vi "Rack Status.vi"(7 "Address":u16, 8 "Error In":errorcluster, 11 "VISA Resource in":refnum<visa-resource-name>) -> (0 "Error Out":errorcluster, 1 "Rack Status Cluster":T1, 2 "Rack Status":u8 format="%.0b", 3 "VISA Resource out":refnum<visa-resource-name>)   [LabVIEW 2015, in "KIT QV.lvlib"]
doc: "Read rack status. It's the OR/AND of all marked detectors including status of control mode."
uses:
  KIT QV.lvlib
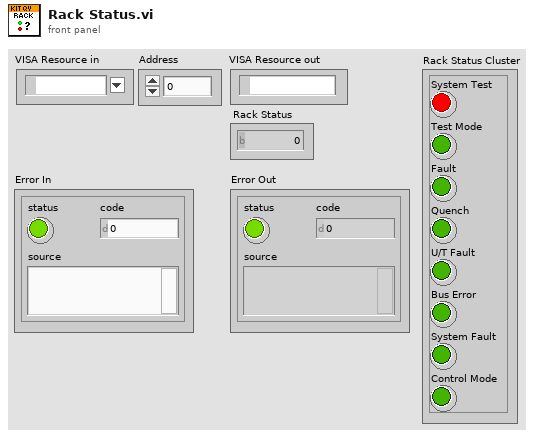
[diagram p1: front panel]
types:
  T1 = cluster{"System Test":bool, "Test Mode":bool, "Fault":bool, "Quench":bool, "U/T Fault":bool, "Bus Error":bool, "System Fault":bool, "Control Mode":bool}
  T2 = cluster{"Boolean array[0]":bool, "Boolean array[1]":bool, "Boolean array[2]":bool, "Boolean array[3]":bool, "Boolean array[4]":bool, "Boolean array[5]":bool, "Boolean array[6]":bool, "Boolean array[7]":bool}
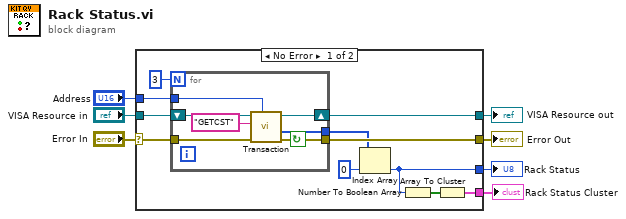
[diagram p0: block diagram]
diagram:
  n1 = case shown="No Error" "Error In" {
    selector: "Error In" -> [w17 w26]
    tunnel: [w15 w27] -> w7
    tunnel: [w14 w26] -> w6
    tunnel: "VISA Resource in" -> [w18 w27]
    tunnel: "Address" -> [w16 _]
    tunnel: [w11 _] -> w2
    tunnel: [w9 _] -> w1
    frame No Error {
      n2 = for {
        N: 3 -> [_]
        tunnel: w16 -> [w22]
        tunnel: [w20] -> w13
        shift-right: [w21] -> w15
        shift-left: w18 -> [w25]
        tunnel: w17 -> [w24]
        tunnel: [w19] -> w14
        stop <- w19 continue-if-true
        n3 = call "Transaction.vi"("Address"=w22, "error in (no error)"=w24, "Command"="GETCST" ("Reset Command"), "VISA Resource in"=w25) -> ("error out"=w19:errorcluster, "Parameter out"=w20:u8[], "VISA Resource out"=w21:refnum<visa-resource-name>)  [unwired: 5 in]
      }
      n4 = Index Array(array=w13, index=0) -> (element=w11:u8)
      n5 = Number To Boolean Array(number=w11) -> (Boolean array=w10:bool[])
      n6 = Array To Cluster(array=w10) -> (cluster=w9:T2)
    }
    frame Error {
    }
  }
  "Error Out" <- w6
  "VISA Resource out" <- w7
  "Rack Status" <- w2
  "Rack Status Cluster" <- w1
